vi "A14rowin.vi"(0 "Basic Size":dbl, 5 "error in (no error)":errorcluster) -> (6 "Row":i32, 8 "error out":errorcluster)   [LabVIEW 2023]
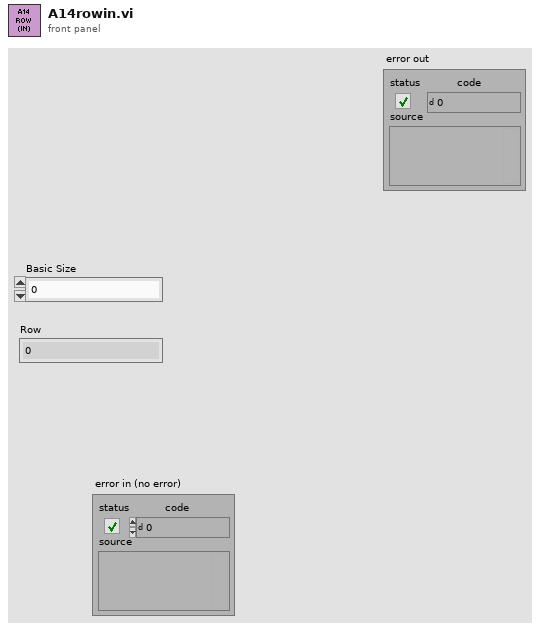
[diagram p1: front panel]
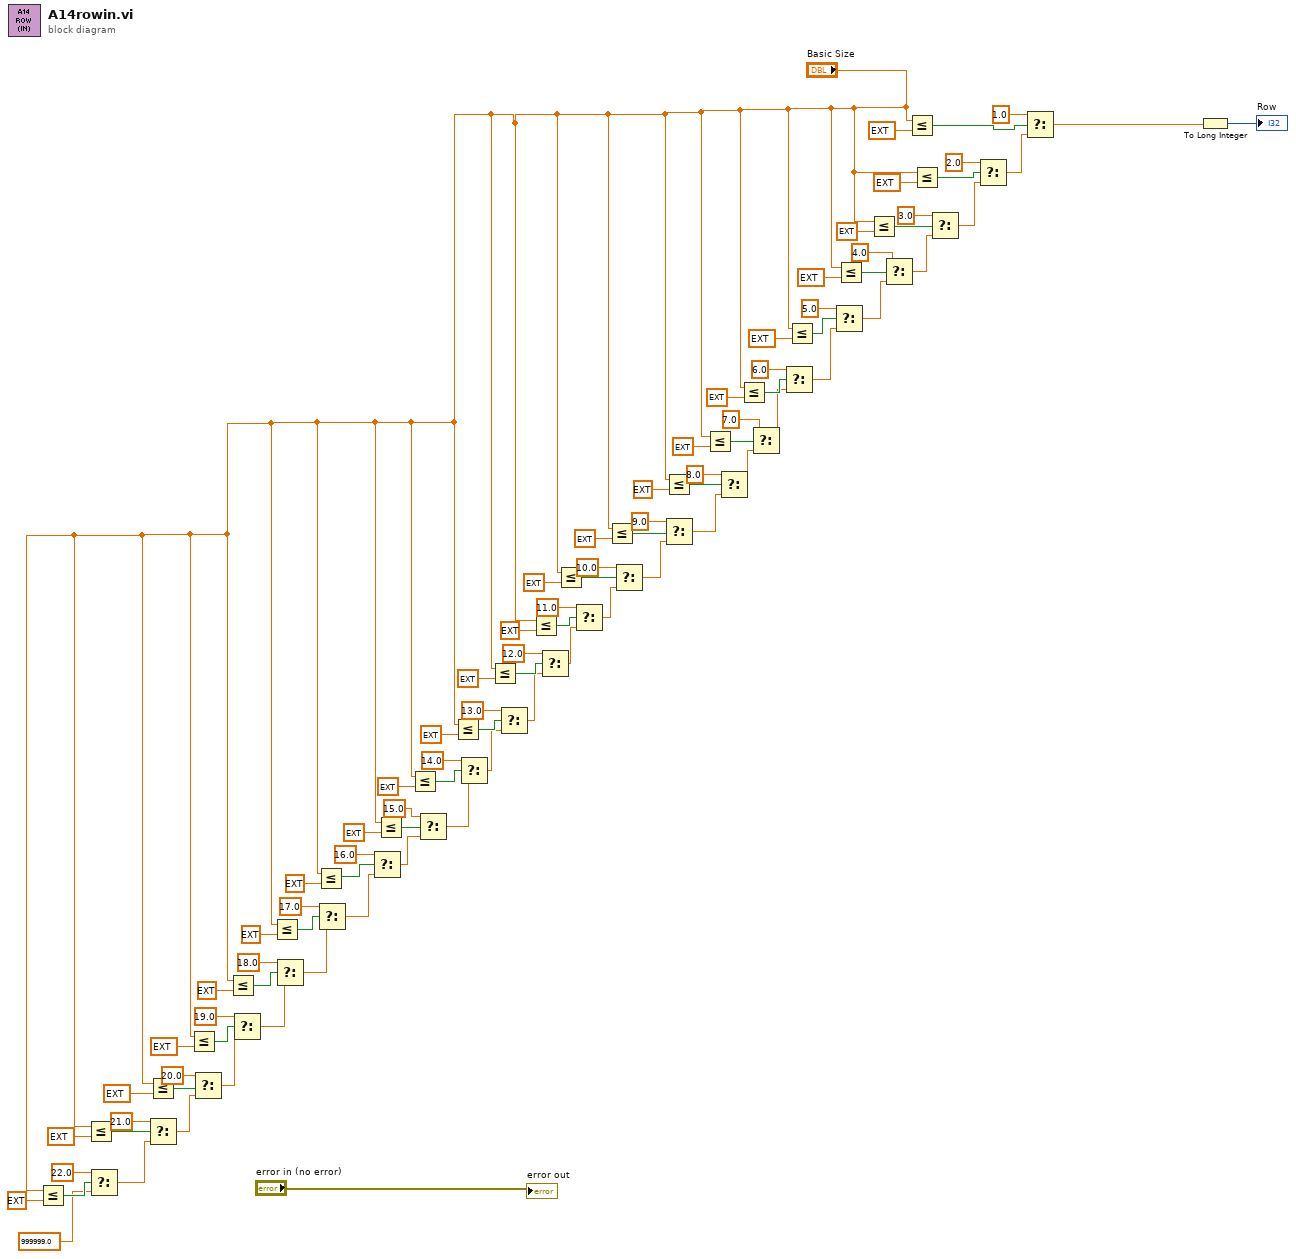
[diagram p0: block diagram]
diagram:
  n1 = Less Or Equal?(x="Basic Size", y=ext 16.0) -> (x <= y?=w6:bool)
  n2 = Less Or Equal?(x="Basic Size", y=ext 14.2) -> (x <= y?=w10:bool)
  n3 = Select(t=22.0, s=w6, f=999999.0) -> (s? t:f=w8:dbl)
  n4 = Less Or Equal?(x="Basic Size", y=ext 12.6000000000000000003) -> (x <= y?=w15:bool)
  n5 = Select(t=21.0, s=w10, f=w8) -> (s? t:f=w13:dbl)
  n6 = Less Or Equal?(x="Basic Size", y=ext 11.2) -> (x <= y?=w18:bool)
  n7 = Select(t=20.0, s=w15, f=w13) -> (s? t:f=w16:dbl)
  n8 = Less Or Equal?(x="Basic Size", y=ext 10.0) -> (x <= y?=w22:bool)
  n9 = Select(t=19.0, s=w18, f=w16) -> (s? t:f=w20:dbl)
  n10 = Less Or Equal?(x="Basic Size", y=ext 9.0) -> (x <= y?=w26:bool)
  n11 = Select(t=18.0, s=w22, f=w20) -> (s? t:f=w24:dbl)
  n12 = Less Or Equal?(x="Basic Size", y=ext 8.0) -> (x <= y?=w30:bool)
  n13 = Select(t=17.0, s=w26, f=w24) -> (s? t:f=w28:dbl)
  n14 = Select(t=16.0, s=w30, f=w28) -> (s? t:f=w32:dbl)
  n15 = Less Or Equal?(x="Basic Size", y=ext 7.2) -> (x <= y?=w34:bool)
  n16 = Less Or Equal?(x="Basic Size", y=ext 6.4) -> (x <= y?=w38:bool)
  n17 = Select(t=15.0, s=w34, f=w32) -> (s? t:f=w36:dbl)
  n18 = Less Or Equal?(x="Basic Size", y=ext 5.6) -> (x <= y?=w42:bool)
  n19 = Select(t=14.0, s=w38, f=w36) -> (s? t:f=w40:dbl)
  n20 = Less Or Equal?(x="Basic Size", y=ext 4.8000000000000000002) -> (x <= y?=w46:bool)
  n21 = Select(t=13.0, s=w42, f=w40) -> (s? t:f=w44:dbl)
  n22 = Less Or Equal?(x="Basic Size", y=ext 4.0) -> (x <= y?=w50:bool)
  n23 = Select(t=12.0, s=w46, f=w44) -> (s? t:f=w48:dbl)
  n24 = Less Or Equal?(x="Basic Size", y=ext 3.2) -> (x <= y?=w54:bool)
  n25 = Select(t=11.0, s=w50, f=w48) -> (s? t:f=w52:dbl)
  n26 = Less Or Equal?(x="Basic Size", y=ext 2.5999999999999999999) -> (x <= y?=w58:bool)
  n27 = Select(t=10.0, s=w54, f=w52) -> (s? t:f=w56:dbl)
  n28 = Less Or Equal?(x="Basic Size", y=ext 2.0) -> (x <= y?=w62:bool)
  n29 = Select(t=9.0, s=w58, f=w56) -> (s? t:f=w60:dbl)
  n30 = Less Or Equal?(x="Basic Size", y=ext 1.6) -> (x <= y?=w66:bool)
  n31 = Select(t=8.0, s=w62, f=w60) -> (s? t:f=w64:dbl)
  n32 = Less Or Equal?(x="Basic Size", y=ext 1.20000000000000000004) -> (x <= y?=w70:bool)
  n33 = Select(t=7.0, s=w66, f=w64) -> (s? t:f=w68:dbl)
  n34 = Select(t=6.0, s=w70, f=w68) -> (s? t:f=w72:dbl)
  n35 = Less Or Equal?(x="Basic Size", y=ext 0.96) -> (x <= y?=w74:bool)
  n36 = Select(t=5.0, s=w74, f=w72) -> (s? t:f=w76:dbl)
  n37 = Less Or Equal?(x="Basic Size", y=ext 0.72000000000000000003) -> (x <= y?=w79:bool)
  n38 = Less Or Equal?(x="Basic Size", y=ext 0.4) -> (x <= y?=w83:bool)
  n39 = Select(t=4.0, s=w79, f=w76) -> (s? t:f=w80:dbl)
  n40 = Less Or Equal?(x="Basic Size", y=ext 0.12) -> (x <= y?=w87:bool)
  n41 = Less Or Equal?(x="Basic Size", y=ext 0.24) -> (x <= y?=w86:bool)
  n42 = Select(t=3.0, s=w83, f=w80) -> (s? t:f=w84:dbl)
  n43 = Select(t=2.0, s=w86, f=w84) -> (s? t:f=w91:dbl)
  n44 = Select(t=1.0, s=w87, f=w91) -> (s? t:f=w90:dbl)
  n45 = To Long Integer(number=w90) -> (32bit integer=→"Row":i32)
  "error out" <- "error in (no error)"
